vi "ActionVIOnCompile.vi"(8 "error in (no error)":errorcluster, 11 "Device Item Ref in":T1 format="%.0x") -> (0 "error out":errorcluster)   [LabVIEW 2017, in "Routing and Faulting System Explorer.lvlib"]
uses:
  Routing and Faulting System Explorer.lvlib
  <vilib>/NI Veristand/Custom Device API/Custom Device Item Ref.ctl
  Shared/Compiled.Settings.ctl
  Shared/Communication Configuration.ctl
  Shared/Routing and Faulting Configuration.ctl
  Shared/Routing Channel Configuration.ctl
  Shared/Value-Connections Map.ctl
  Shared/Connection.ctl
  Shared/Alias Mapping.ctl
  Shared/FIFO Indices.ctl
  Shared/Constants.vi
  Get Channel Data in By Channel ID.vi
  <vilib>/NI Veristand/Custom Device API/Set Item Property (Variant).vi
  <vilib>/NI Veristand/Custom Device API/Custom Device API.lvlib
  Shared/Routing and Faulting Shared.lvlib
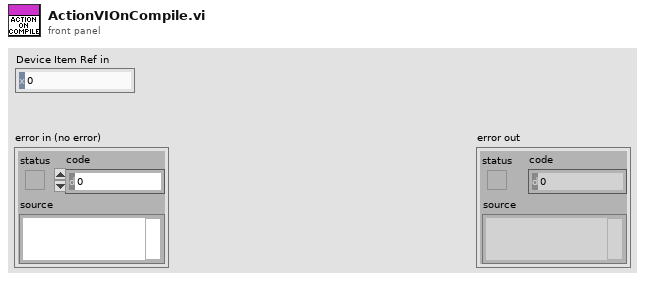
[diagram p1: front panel]
types:
  T1 = typedef "Custom Device API.lvlib/Custom Device Item Ref.ctl" = u64
  T2 = typedef "Routing and Faulting Shared.lvlib/FIFO Indices.ctl" = cluster{"Status Channel":i32, "Heartbeat Channel":i32}
  T3 = typedef "Routing and Faulting Shared.lvlib/Compiled.Settings.ctl" = cluster{"Custom Device Name":string, "Communication Configuration":T4, "Routing and Faulting Configuration":T5, "Status Channels FIFO Indices":T2}
  T4 = typedef "Routing and Faulting Shared.lvlib/Communication Configuration.ctl" = cluster{"Consumer Queue Names":string[]}
  T5 = typedef "Routing and Faulting Shared.lvlib/Routing and Faulting Configuration.ctl" = cluster{"Routing Channel Configurations":T6[], "Alias Mappings":T9[]}
  T6 = typedef "Routing and Faulting Shared.lvlib/Routing Channel Configuration.ctl" = cluster{"Channel Name":string, "Initial Value":dbl, "FIFO Index":i32, "Value-Connections Map":T7}
  T7 = typedef "Routing and Faulting Shared.lvlib/Value-Connections Map.ctl" = cluster{"State Value Array":i32[], "Connection List Array":cluster{"Connection List":T8[]}[]}
  T8 = typedef "Routing and Faulting Shared.lvlib/Connection.ctl" = cluster{"Resource":string, "Source":string, "Destination":string}
  T9 = typedef "Routing and Faulting Shared.lvlib/Alias Mapping.ctl" = cluster{"Endpoint":string, "Alias":string}
  T10 = typedef "Custom Device API.lvlib/Custom Device Item Info.ctl" = cluster{"Name":string, "Is Channel":bool, "GUID":string, "Is Waveform":bool}
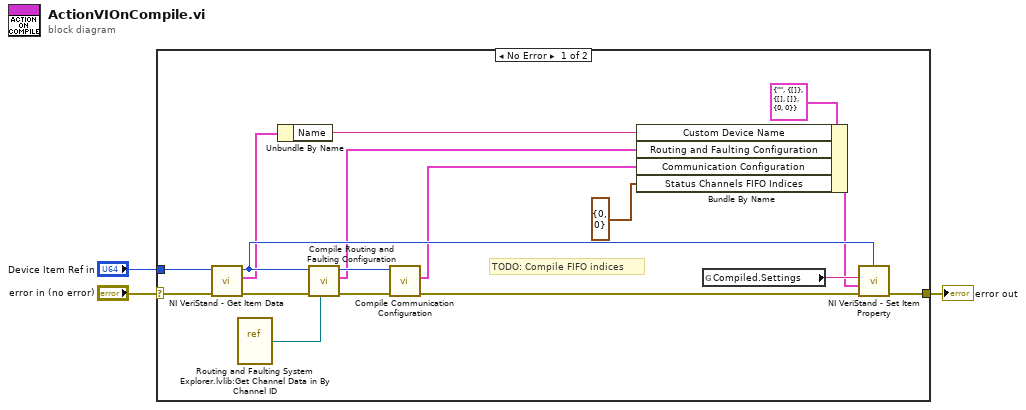
[diagram p0: block diagram]
diagram:
  n1 = case shown="No Error" "error in (no error)" {
    selector: "error in (no error)" -> [w19 w21]
    tunnel: [w20 w21] -> w2
    tunnel: "Device Item Ref in" -> [w18 _]
    frame No Error {
      # "TODO: Compile FIFO indices"
      n2 = call <vilib>:"NI VeriStand - Get Item Data.vi"("error in (no error)"=w19, "Item Ref in"=w18) -> ("error out"=w12:errorcluster, "Item Info"=w7:T10, "Item Ref out"=w15:T1)  [unwired: 6 in, 1 out]
      n3 = vi-ref "Routing and Faulting System Explorer.lvlib:Get Channel Data in By Channel ID.vi"() -> (w6:refnum<vi>)
      n4 = Unbundle By Name(w7) -> ("Name"=w10:string)
      n5 = call "Compile Routing and Faulting Configuration.vi"("Get Channel Data Refnum"=w6, "error in (no error)"=w12, "Device Ref in"=w15) -> ("error out"=w13:errorcluster, "RaF Configuration"=w9:T5, "Device Ref out"=w14:T1)  [unwired: 6 in]
      n6 = call "Compile Communication Configuration.vi"("error in (no error)"=w13, "Device Ref in"=w14) -> ("error out"=w11:errorcluster, "Communication Configuration"=w5:T4)  [unwired: 7 in, 1 out]
      n7 = Bundle By Name(cluster=T3 {"Custom Device Name"="", "Communication Configuration"={"Consumer Queue Names"=[]}, "Routing and Faulting Configuration"={"Routing Channel Configurations"=[], "Alias Mappings"=[]}, "Status Channels FIFO Indices"={"Status Channel"=0, "Heartbeat Channel"=0}} ("Compiled.Settings.ctl"), "Custom Device Name"=w10, "Routing and Faulting Configuration"=w9, "Communication Configuration"=w5, "Status Channels FIFO Indices"=T2 {"Status Channel"=0, "Heartbeat Channel"=0}) -> (w4:T3)
      n8 = global read "Constants.vi" "Compiled.Settings"() -> (w16:string)
      n9 = call-poly <vilib>:"NI VeriStand - Set Item Property.vi"("error in (no error)"=w11, "Value"=w4, "Property Name"=w16, "Item Ref in"=w15) -> ("error out"=w20:errorcluster)  [unwired: 5 in, 2 out]
    }
    frame Error {
    }
  }
  "error out" <- w2
